vi "sort_according_to_x.vi"(8 "error in (no error)":errorcluster, 10 "points in":refnum<class "SpaceVector.lvclass">[](array[class])) -> (0 "error out":errorcluster, 2 "points out":refnum<class "SpaceVector.lvclass">[](array[class]))   [LabVIEW 2010, in "TrajectoryDL120126ArbitraryLine2D.lvclass"]
uses:
  TrajectoryDL120126ArbitraryLine2D.lvclass
  common/classes/SpaceVector/SpaceVector/SpaceVector.lvclass
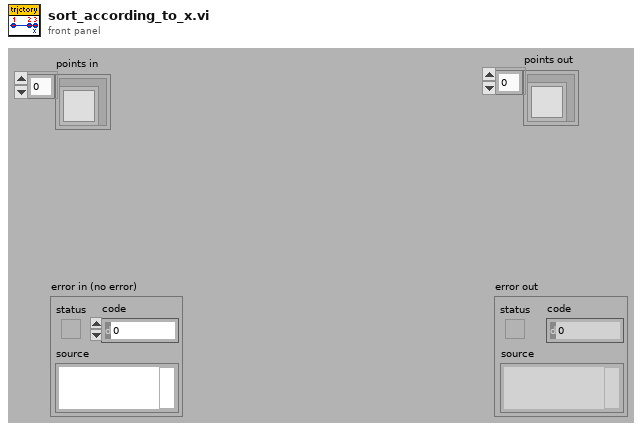
[diagram p1: front panel]
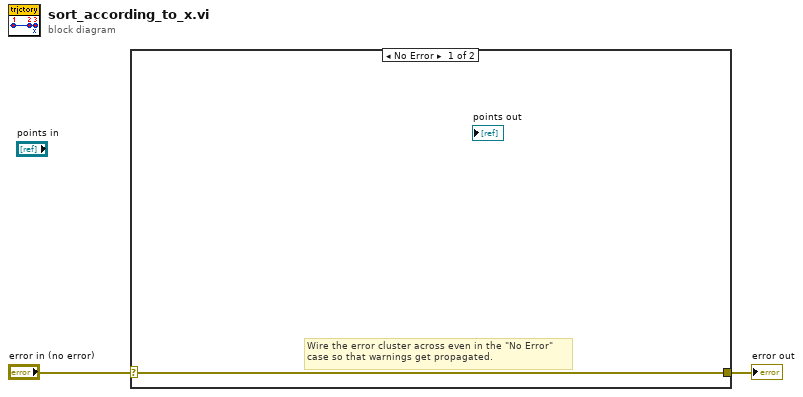
[diagram p0: block diagram]
diagram:
  n1 = case shown="No Error" "error in (no error)" {
    selector: "error in (no error)" -> [w3 w4]
    tunnel: [w3 w4] -> w1
    frame No Error {
      # "Wire the error cluster across even in the \"No Error\"\ncase so that warnings get propagated."
    }
    frame Error {
    }
  }
  "error out" <- w1
